vi "Init_Action.vi"(8 "error in":errorcluster caption="错误输入（无错误）", 11 "AutoDetPort":bool) -> (0 "error out":errorcluster caption="错误输出")   [LabVIEW 2013]
uses:
  SystemCode/SysControl/Slot.ctl
  GlobalValue.vi
  <vilib>/Utility/error.llb/Error Cluster From Error Code.vi
  <vilib>/ErrorRing/Error Ring.xnode
  <resource>/objmgr/daqmx.rc
  InstrumentDrivers/USB-CAN/InitConfig.ctl
  InstrumentDrivers/USB-CAN/DevType.ctl
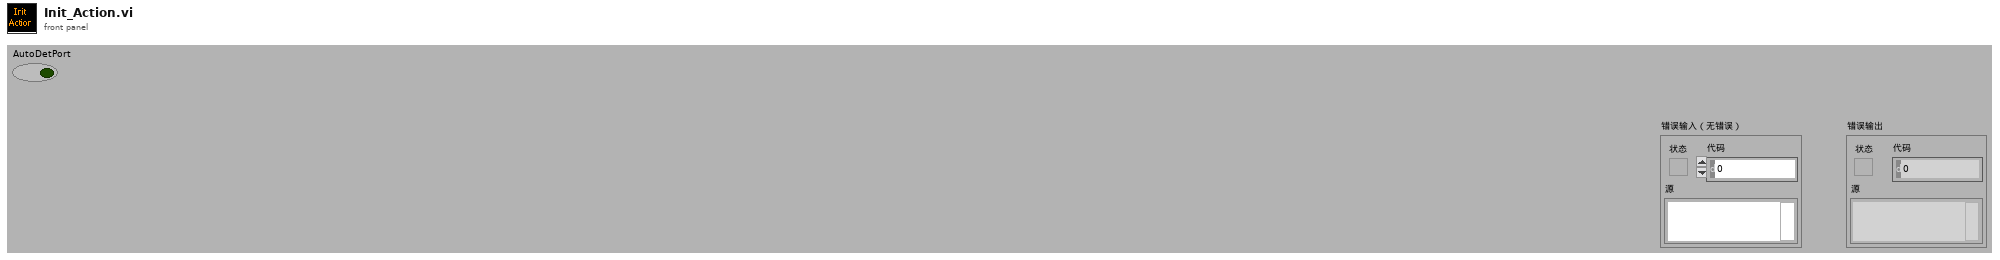
[diagram p1: front panel]
types:
  T1 = typedef "Slot.ctl" = enum16{"Slot1", "Slot2", "Slot3", "Slot4"}
  T2 = typedef "InitConfig.ctl" = cluster{"AccCode":u32, "AccMask":u32, "Reserved":u32, "Filter":u8, "kCanBaud":u8, "Timing0":u8, "Timing1":u8, "Mode":u8, "CanRx_IER":u8}
  T3 = typedef "DevType.ctl" = u16
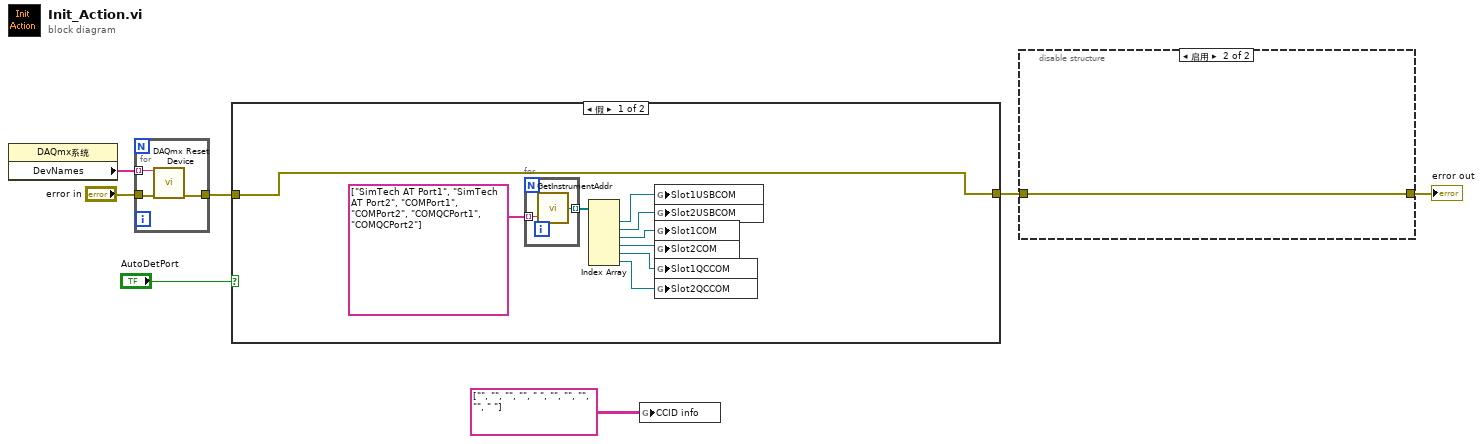
[diagram p0: block diagram]
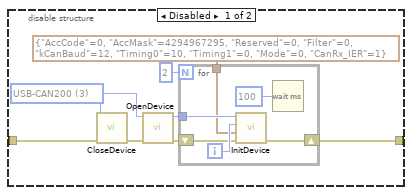
[diagram p2: hidden frame]
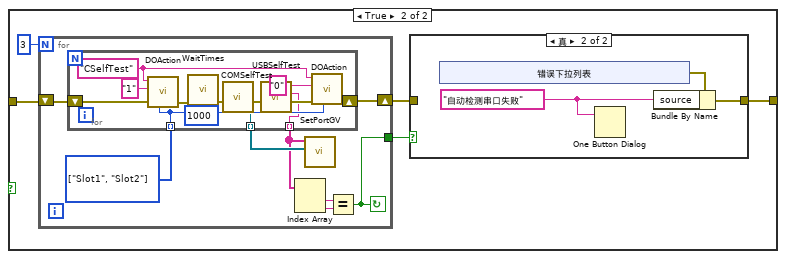
[diagram p3: hidden frame]
diagram:
  n1 = property class="DAQmx系统"() -> ("DevNames"=w6:tag[])  [unwired: 2 in, 2 out]
  n2 = for {
    tunnel: [w9] -> w5
    tunnel: "error in" -> [w10]
    tunnel: w6 -> [w8] mode=indexing
    n3 = call <vilib>:"DAQmx Reset Device.vi"("device in"=w8, "error in"=w10) -> ("error out"=w9:errorcluster)  [unwired: 13 in]
  }
  n4 = case shown="假" "AutoDetPort" {
    tunnel: w5 -> [w13 w26]
    tunnel: [w13 w25] -> w3
    frame False {
      n5 = for {
        tunnel: string[] ["SimTech AT Port1", "SimTech AT Port2", "COMPort1", "COMPort2", "COMQCPort1", "COMQCPort2"] ("数组") -> [w21] mode=indexing
        tunnel: [w20] -> w18 mode=indexing
        n6 = call "GetInstrumentAddr.vi"("String"=w21) -> ("VISA session"=w20:refnum<visa-resource-name>)  [unwired: 1 out]
      }
      n7 = Index Array(array=w18) -> (element #1=w17:refnum<visa-resource-name>, element #2=w16:refnum<visa-resource-name>, element #3=w15:refnum<visa-resource-name>, element #4=w14:refnum<visa-resource-name>, element #5=w12:refnum<visa-resource-name>, element #6=w11:refnum<visa-resource-name>)  [unwired: 6 in]
      n8 = global write "GlobalValue.vi" "Slot1USBCOM"(w17) -> ()
      n9 = global write "GlobalValue.vi" "Slot2USBCOM"(w16) -> ()
      n10 = global write "GlobalValue.vi" "Slot1COM"(w15) -> ()
      n11 = global write "GlobalValue.vi" "Slot2COM"(w14) -> ()
      n12 = global write "GlobalValue.vi" "Slot1QCCOM"(w12) -> ()
      n13 = global write "GlobalValue.vi" "Slot2QCCOM"(w11) -> ()
    }
    frame True {
      n14 = for {
        N: 3 -> [_]
        shift-right: [w39] -> w22
        shift-left: w26 -> [w40]
        tunnel: [w35] -> w23
        stop <- w35 continue-if-true
        w42 = T1[] [enum."Slot1", enum."Slot2"] items=["Slot1", "Slot2", "Slot3", "Slot4"]
        n15 = for {
          tunnel: w42 -> [w53] mode=indexing
          shift-right: [w50] -> w39
          shift-left: w40 -> [w51]
          tunnel: [w49] -> w41 mode=indexing
          tunnel: [w46] -> w38 mode=indexing
          w52 = "CSelfTest" ("CH")
          n16 = call "DOAction.vi"("Slot"=w53, "error in"=w51, "State"="1", "CH"=w52) -> ("error out"=w45:errorcluster)  [unwired: 7 in]
          n17 = call "WaitTimes.vi"("WaitTimes"=u32 1000, "error in (no error)"=w45) -> ("error out"=w44:errorcluster)  [unwired: 9 in]
          n18 = call "COMSelfTest.vi"("error in (no error)"=w44) -> ("error out"=w48:errorcluster, "COMOUT"=w49:refnum<visa-resource-name>)  [unwired: 9 in]
          n19 = call "USBSelfTest.vi"("error in (no error)"=w48) -> ("error out"=w47:errorcluster, "USB"=w46:string)  [unwired: 8 in, 1 out]
          n20 = call "DOAction.vi"("Slot"=w53, "error in"=w47, "State"="0", "CH"=w52) -> ("error out"=w50:errorcluster)  [unwired: 7 in]
        }
        n21 = Index Array(array=w38) -> (element #1=w37:string, element #2=w36:string)  [unwired: 2 in]
        n22 = call "SetPortGV.vi"("COM"=w41, "USB"=w38) -> ()  [unwired: 10 in]
        n23 = Equal?(x=w37, y=w36) -> (x = y?=w35:bool)
      }
      n24 = case shown="真" w23 {
        tunnel: [w27 w28] -> w25
        tunnel: w22 -> [w27 _]
        frame False {
        }
        frame True {
          w29 = "自动检测串口失败" ("消息")
          n25 = xnode "错误下拉列表"() -> ("错误输出"=w30:errorcluster)
          n26 = One Button Dialog(message=w29) -> ()  [unwired: 1 in, 1 out]
          n27 = Bundle By Name(cluster=w30, "source"=w29) -> (w28:errorcluster)
        }
      }
    }
  }
  n28 = global write "GlobalValue.vi" "CCID info"(string[][] [["", "", "", "", " "], ["", "", "", "", " "]] ("CCID info")) -> ()
  n29 = disable-structure shown="启用" {
    disable-tunnel: [w59 w70] -> w4
    disable-tunnel: w3 -> [w58 w70]
    frame Disabled {
      w56 = T3 3 items=["PCI-CAN200"=7, "USB-CAN"=2, "USB-CAN200"=3] ("DeviceType")
      n30 = call "CloseDevice.vi"("错误输入（无错误）"=w58, "DeviceType"=w56) -> ("错误输出"=w57:errorcluster)  [unwired: 7 in, 2 out]
      n31 = call "OpenDevice.vi"("错误输入（无错误）"=w57, "DeviceType"=w56) -> ("错误输出"=w61:errorcluster, "DeviceTypeOut"=w63:u16)  [unwired: 7 in, 1 out]
      n32 = for {
        N: 2 -> [_]
        tunnel: w63 -> [w69]
        shift-right: [w65] -> w59
        shift-left: w61 -> [w66]
        tunnel: T2 {"AccCode"=0, "AccMask"=4294967295, "Reserved"=0, "Filter"=0, "kCanBaud"=12, "Timing0"=10, "Timing1"=0, "Mode"=0, "CanRx_IER"=1} ("InitConfig") -> [w64]
        i -> [w68]
        n33 = call "InitDevice.vi"("错误输入（无错误）"=w66, "InitConfig"=w64, "CanChannel"=w68, "DeviceType"=w69) -> ("错误输出"=w65:errorcluster)  [unwired: 5 in, 2 out]
        n34 = Wait (ms)(milliseconds to wait=u32 100 ("等待时间（毫秒）")) -> ()  [unwired: 1 out]
      }
    }
    frame Enabled {
    }
  }
  "error out" <- w4
